vi "Delay.vi"(8 "error in (no error)":errorcluster, 10 "Delay Value (150)":i32=150, 11 "VISA resource name":refnum<visa-resource-name>) -> (0 "error out":errorcluster, 3 "VISA resource name out":refnum<visa-resource-name>)   [LabVIEW 2019, in "BK Precision 1823A.lvlib"]
doc: "This VI functions as a delay. <b>Delay Value</b> input defines the delay time in milliseconds (ms)."
uses:
  BK Precision 1823A.lvlib
panel:
  # "(c) 2009 B&K PRECISION CORPORATION.  ALL RIGHTS RESERVED."
  # "ms"
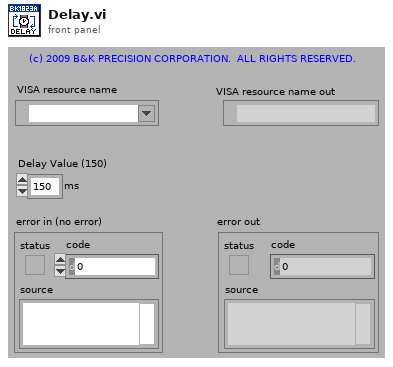
[diagram p1: front panel]
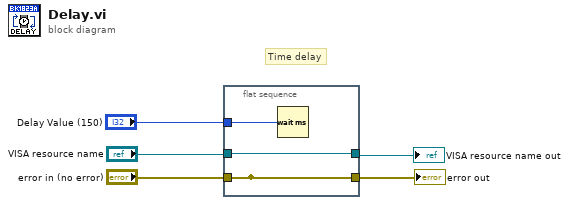
[diagram p0: block diagram]
diagram:
  # "Time delay"
  n1 = flat-sequence {
    tunnel: "VISA resource name" -> [w8]
    tunnel: [w7] -> _
    tunnel: [w7] -> w2
    tunnel: [w8] -> w5
    tunnel: "error in (no error)" -> [w7]
    tunnel: "Delay Value (150)" -> [w6]
    frame #0 {
      n2 = Wait (ms)(milliseconds to wait=w6) -> ()  [unwired: 1 out]
    }
  }
  "VISA resource name out" <- w5
  "error out" <- w2
